vi "Double Array.vi"(8 "Error In":errorcluster) -> (0 "Error Out":errorcluster)   [LabVIEW 2018, in "Tests.lvlib" / "From Msgpack.lvlib"]
uses:
  From Msgpack.lvlib
  <vilib>/addons/_JKI Toolkits/Caraya/classes/Test/Test.lvclass
  src/Toolkit/Toolkit.lvlib
  <vilib>/addons/_JKI Toolkits/Caraya/classes/Assert/Assert.lvclass
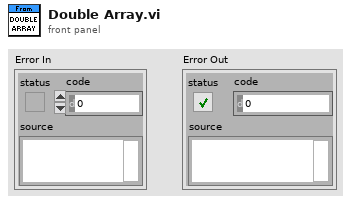
[diagram p1: front panel]
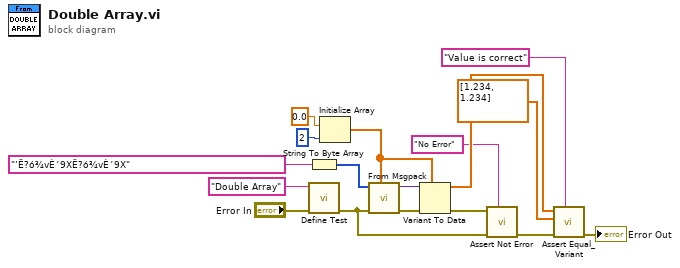
[diagram p0: block diagram]
diagram:
  n1 = String To Byte Array(string="’Ë?ó¾vÈ´9XË?ó¾vÈ´9X") -> (unsigned byte array=w14:u8[])
  n2 = call <vilib>:"Define Test.vi"("error in (no error)"="Error In", "Label (VI Title)"="Double Array") -> ("error out"=w11:errorcluster)  [unwired: 9 in]
  n3 = Initialize Array(0.0, 2 ("dimension size")) -> (w1:dbl[])
  n4 = call "From Msgpack.vi"("Types and Defaults"=w1, "Error In"=w11, "Msgpack Data"=w14) -> ("Error Out"=w15:errorcluster, "Value"=w13:variant)  [unwired: 7 in]
  n5 = Variant To Data(error in=w15, type=w1, Variant=w13) -> (data=w8:dbl[], error out=w12:errorcluster)
  n6 = call <vilib>:"Assert Not Error.vi"("Label"="No Error", "error in (no error)"=w11, "Not Error?"=w12) -> ("error out"=w10:errorcluster)  [unwired: 8 in]
  n7 = call <vilib>:"Assert Equal_Variant.vi"("Label"="Value is correct", "error in (no error)"=w10, "Y"=dbl[] [1.234, 1.234], "X"=w8) -> ("error out"=→"Error Out":errorcluster)  [unwired: 7 in]
